vi "LogSpace.vi"(0 "Start":dbl, 1 "Base":dbl=2.0, 2 "Stop":dbl, 3 "Step":dbl) -> (6 "Array":dbl[](array[numeric]), 7 "error out":errorcluster)   [LabVIEW 2020]
uses:
  LinSpace (x0-dx-npts).vi
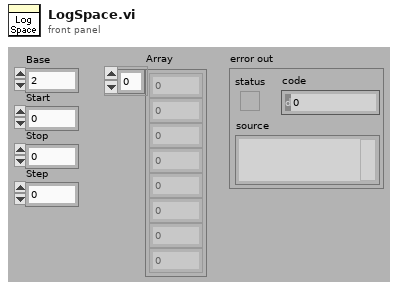
[diagram p1: front panel]
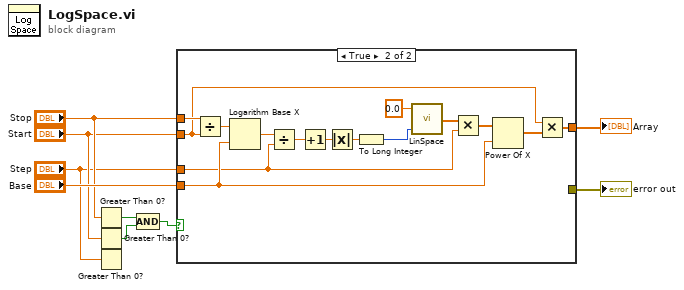
[diagram p0: block diagram]
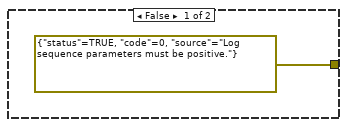
[diagram p2: hidden frame]
diagram:
  n1 = Greater Than 0?(x="Stop") -> (x > 0?=w4:bool)
  n2 = Greater Than 0?(x="Start") -> (x > 0?=w3:bool)
  n3 = Greater Than 0?(x="Step") -> ()  [unwired: 1 out]
  n4 = Compound Arithmetic op=AND(w4, w3) -> (w2:bool)
  n5 = case shown="True" w2 {
    tunnel: [_ w20] -> w9
    tunnel: "Base" -> [_ w15]
    tunnel: "Stop" -> [_ w13]
    tunnel: "Start" -> [_ w12]
    tunnel: "Step" -> [_ w11]
    tunnel: [errorcluster {"status"=TRUE, "code"=0, "source"="Log sequence parameters must be positive."} ("error out") _] -> w1
    frame False {
    }
    frame True {
      n6 = Divide(x=w13, y=w12) -> (x/y=w16:dbl)
      n7 = Logarithm Base X(1:w15, 2:w16) -> (0:w14:dbl)
      n8 = Divide(x=w14, y=w11) -> (x/y=w19:dbl)
      n9 = Increment(x=w19) -> (x+1=w17:dbl)
      n10 = Absolute Value(x=w17) -> (abs(x)=w24:dbl)
      n11 = To Long Integer(number=w24) -> (32bit integer=w23:i32)
      n12 = call-poly "LinSpace.vi"("npts"=w23, "x0"=0.0) -> ("Array"=w22:dbl[])  [unwired: 2 in, 1 out]
      n13 = Multiply(x=w22, y=w11) -> (x*y=w18:dbl[])
      n14 = Power Of X(1:w15, 2:w18) -> (0:w21:dbl[])
      n15 = Multiply(x=w12, y=w21) -> (x*y=w20:dbl[])
    }
  }
  "Array" <- w9
  "error out" <- w1
